vi "Vacuum Test - Step 5.vi"(7 "Step":i32, 8 "error in":errorcluster, 9 "Test Results In":T9, 10 "PAS In":T8 caption="Gas", 11 "Test Configuration":T1) -> (0 "error out":errorcluster, 1 "Test Results Out":T9, 2 "PAS Out":T8 caption="Gas", 3 "Test Configuration Out":T1)   [LabVIEW 2015]
uses:
  CAN Communication/PAS/Typedefs/Session Handle.ctl
  CAN Communication/PAS/PAS.lvclass
  Controls/Test Results.ctl
  Controls/Step Result.ctl
  Controls/Test Configuration.ctl
  Controls/Vacuum Test.ctl
  Controls/Test Timing.ctl
  Controls/Vaccum Thresholds.ctl
  Controls/Helium Test.ctl
  Controls/Helium Thresholds.ctl
  Controls/Functional Test.ctl
  CAN Communication/PAS/Typedefs/Valves.ctl
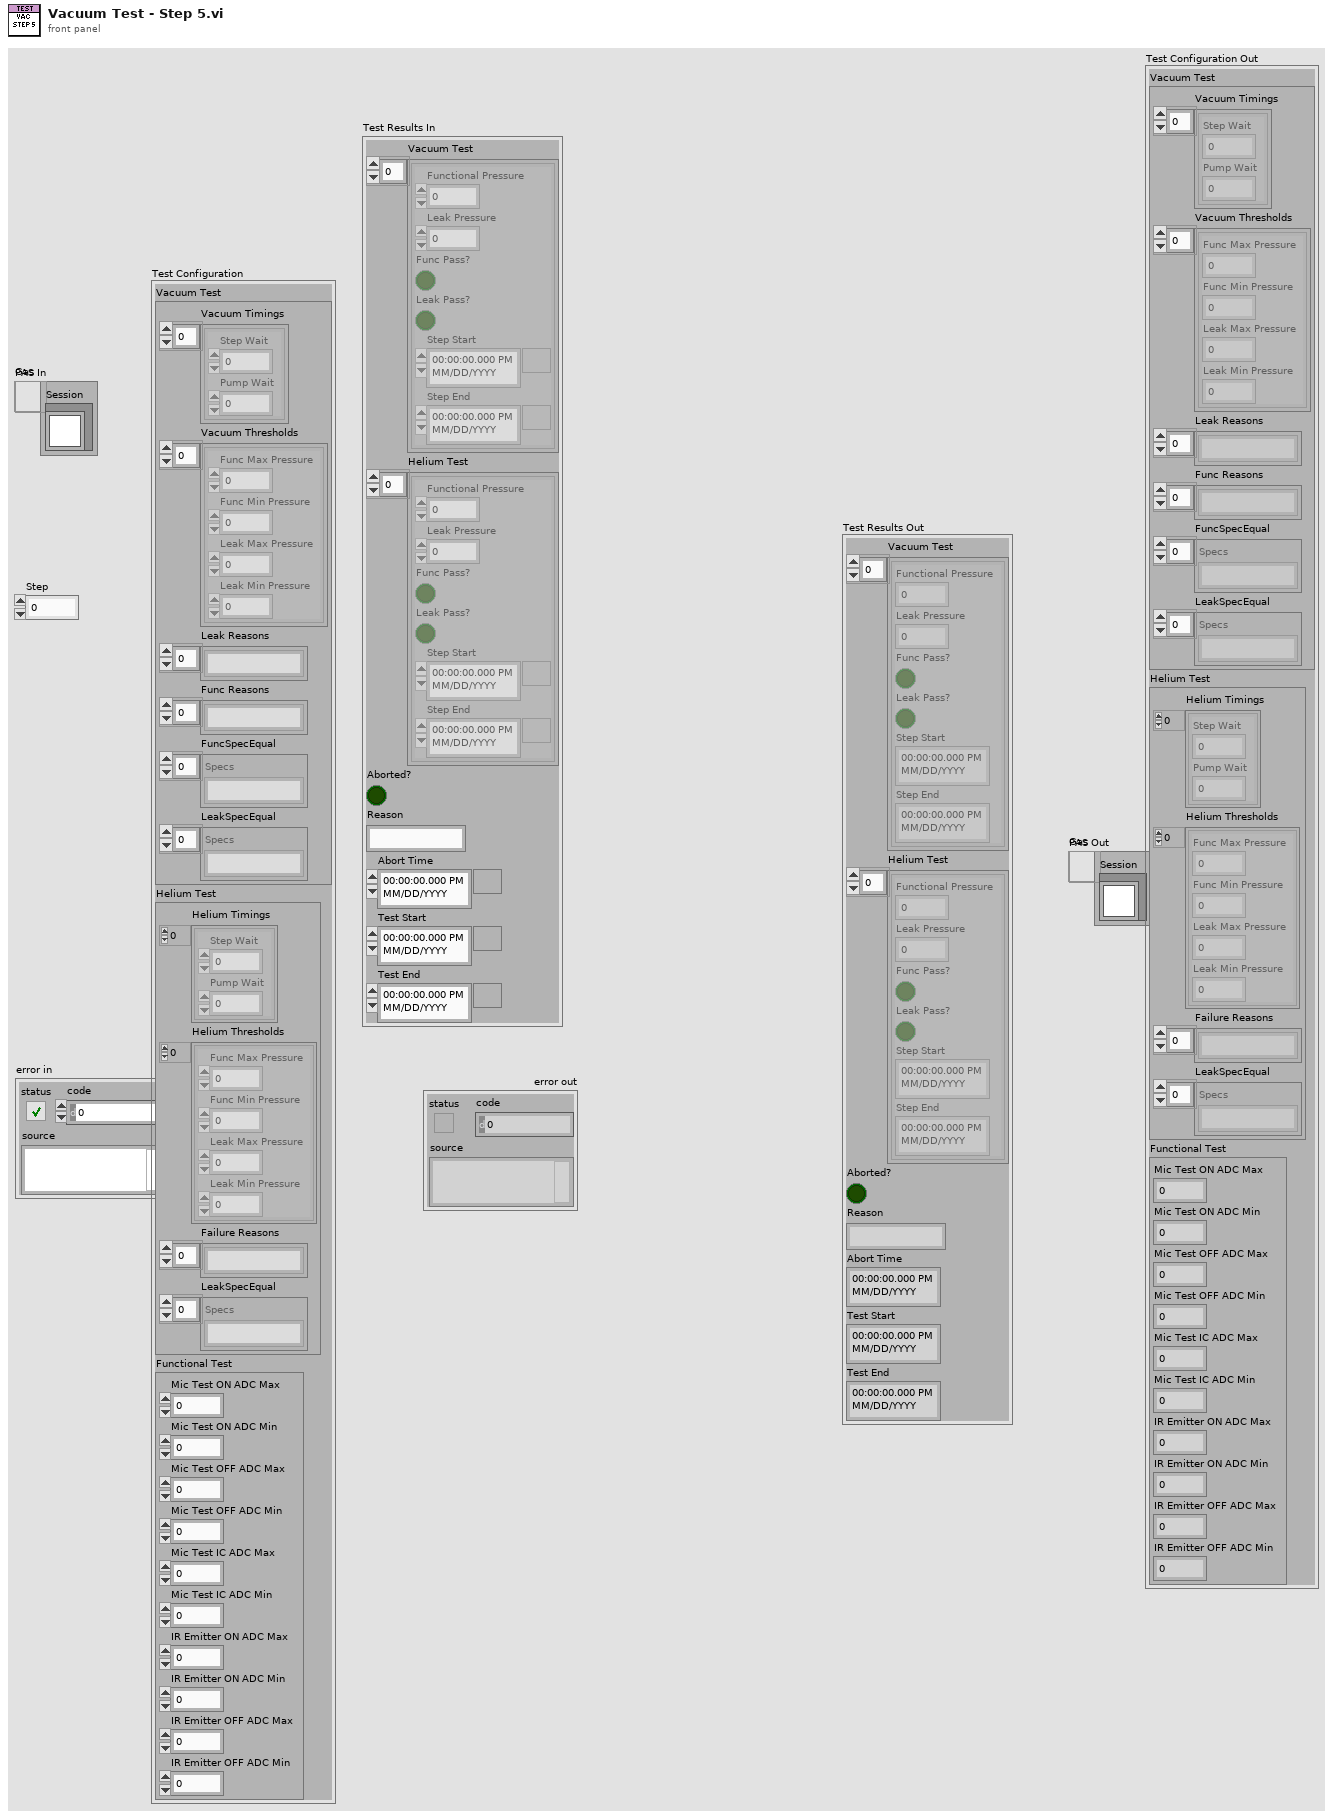
[diagram p1: front panel]
types:
  T1 = typedef "Test Configuration.ctl" = cluster{"Vacuum Test":T2, "Helium Test":T5, "Functional Test":T7}
  T2 = typedef "Vacuum Test.ctl" = cluster{"Vacuum Timings":T3[], "Vacuum Thresholds":T4[], "Leak Reasons":string[], "Func Reasons":string[], "FuncSpecEqual":string[], "LeakSpecEqual":string[]}
  T3 = typedef "Test Timing.ctl" = cluster{"Step Wait":dbl, "Pump Wait":dbl}
  T4 = typedef "Vaccum Thresholds.ctl" = cluster{"Func Max Pressure":dbl, "Func Min Pressure":dbl, "Leak Max Pressure":dbl, "Leak Min Pressure":dbl}
  T5 = typedef "Helium Test.ctl" = cluster{"Helium Timings":T3[], "Helium Thresholds":T6[], "Failure Reasons":string[], "LeakSpecEqual":string[]}
  T6 = typedef "Helium Thresholds.ctl" = cluster{"Func Max Pressure":dbl, "Func Min Pressure":dbl, "Leak Max Pressure":dbl, "Leak Min Pressure":dbl}
  T7 = typedef "Functional Test.ctl" = cluster{"Mic Test ON ADC Max":dbl, "Mic Test ON ADC Min":dbl, "Mic Test OFF ADC Max":dbl, "Mic Test OFF ADC Min":dbl, "Mic Test IC ADC Max":dbl, "Mic Test IC ADC Min":dbl, "IR Emitter ON ADC Max":dbl, "IR Emitter ON ADC Min":dbl, "IR Emitter OFF ADC Max":dbl, "IR Emitter OFF ADC Min":dbl}
  T8 = typedef "PAS.lvclass/Session Handle.ctl" = refnum<data-value>
  T9 = typedef "Test Results.ctl" = cluster{"Vacuum Test":T10[], "Helium Test":T10[], "Aborted?":bool, "Reason":string, "Abort Time":timestamp, "Test Start":timestamp, "Test End":timestamp}
  T10 = typedef "Step Result.ctl" = cluster{"Functional Pressure":dbl, "Leak Pressure":dbl, "Func Pass?":bool, "Leak Pass?":bool, "Step Start":timestamp, "Step End":timestamp}
  T11 = typedef "PAS.lvclass/Valves.ctl" = u16
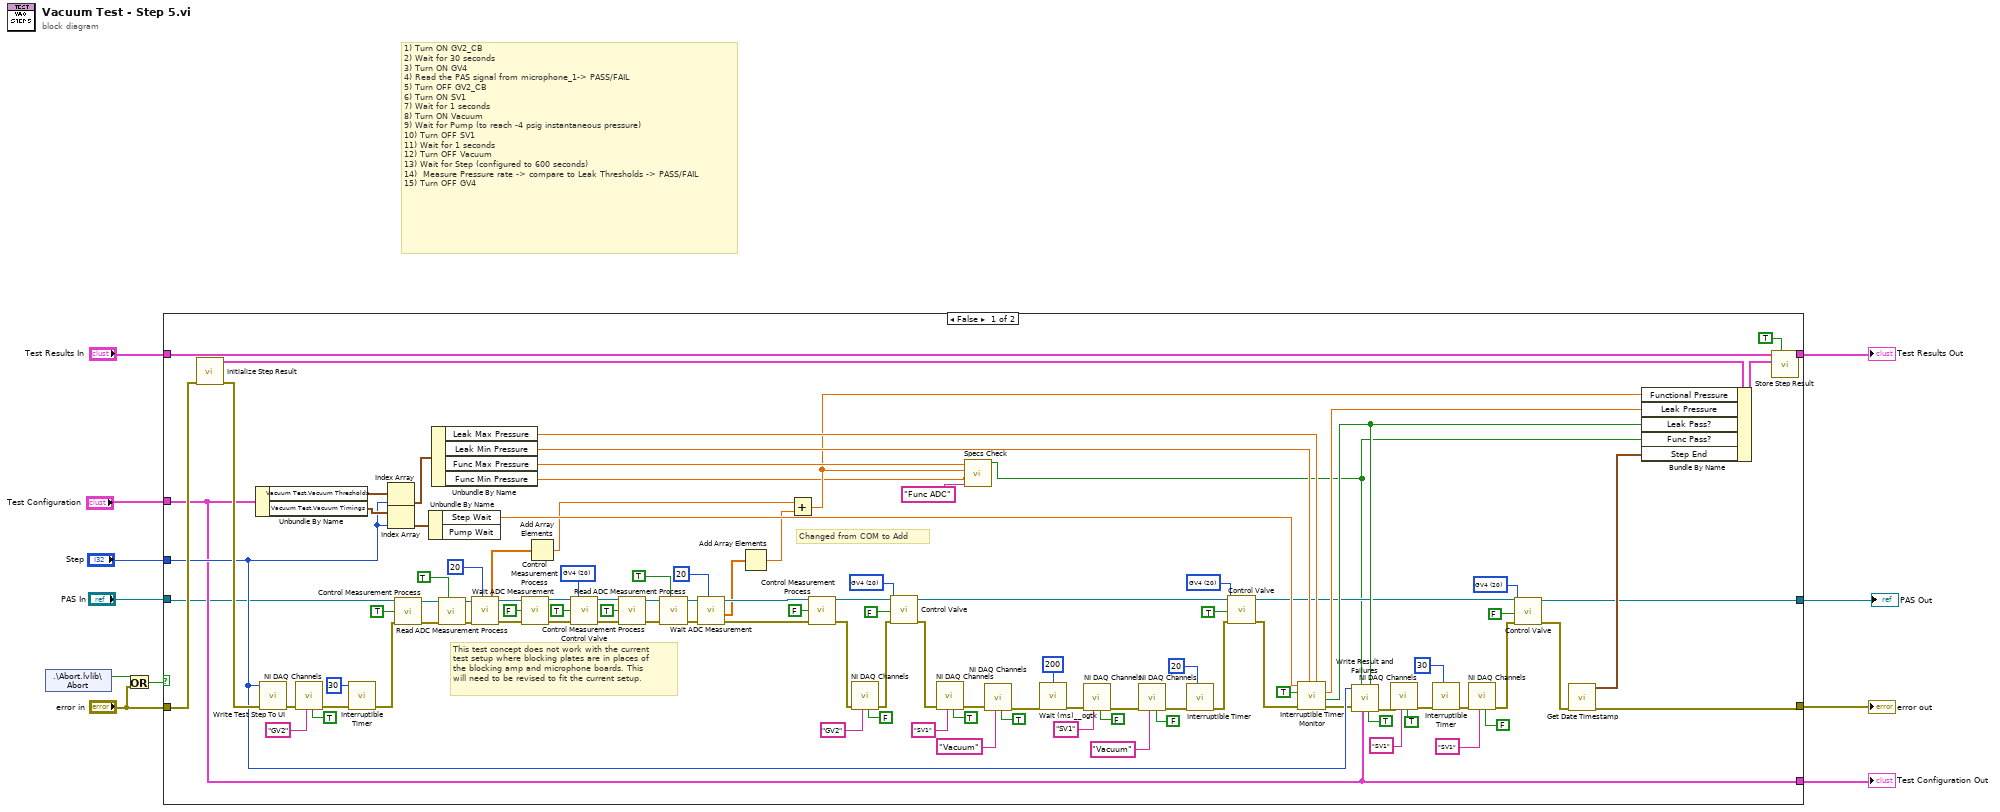
[diagram p0: block diagram]
diagram:
  # "1) Turn ON GV2_CB\n2) Wait for 30 seconds\n3) Turn ON GV4\n4) Read the PAS signal from microphone_1-> PASS/FAIL\n5) Turn OFF GV2_CB\n6) Turn ON SV1\n7) Wait for 1 seconds\n8) Turn ON Vacuum\n9) Wait for Pump (to reach -4 psig instantaneous pressure)\n10) Turn OFF SV1\n11) Wait for 1 seconds\n12) Turn OFF Vacuum\n13) Wait for Step (configured to 600 seconds)\n14)  Measure Pressure rate -> compare to Leak Thresholds -> PASS/FAIL\n15) Turn OFF GV4"
  n1 = shared-variable ".\\Abort.lvlib\\Abort"() -> (w10:bool)  [unwired: 1 in, 1 out]
  n2 = Or(x=w10, y="error in") -> (x .or. y?=w9:bool)
  n3 = case shown="False" w9 {
    tunnel: "error in" -> [w118 w121]
    tunnel: "Test Results In" -> [w115 w122]
    tunnel: [w116 w122] -> w7
    tunnel: [w58 w121] -> w6
    tunnel: "Test Configuration" -> [w99 w120]
    tunnel: "Step" -> [w106 _]
    tunnel: [w99 w120] -> w1
    tunnel: [w93 w119] -> w3
    tunnel: "PAS In" -> [w35 w119]
    frame False {
      w43 = T11 20 items=["GV1"=17, "GV2"=18, "GV3"=19, "GV4"=20] ("Valves")
      w65 = T11 20 items=["GV1"=17, "GV2"=18, "GV3"=19, "GV4"=20] ("Valves")
      w73 = T11 20 items=["GV1"=17, "GV2"=18, "GV3"=19, "GV4"=20] ("Valves")
      w95 = T11 20 items=["GV1"=17, "GV2"=18, "GV3"=19, "GV4"=20] ("Valves")
      # "Changed from COM to Add"
      # "This test concept does not work with the current\ntest setup where blocking plates are in places of\nthe blocking amp and microphone boards. This\nwill need to be revised to fit the current setup."
      n4 = call "Initialize Step Result.vi"("error in (no error)"=w118) -> ("error out"=w117:errorcluster, "New Step Result"=w114:T10)  [unwired: 8 in, 1 out]
      n5 = Unbundle By Name(w99) -> ("Vacuum Test.Vacuum Thresholds"=w111:T4[], "Vacuum Test.Vacuum Timings"=w110:T3[])
      n6 = call "Write Test Step To UI.vi"("error in (no error)"=w117, "Step"=w106) -> ("error out"=w104:errorcluster)  [unwired: 9 in]
      n7 = call "NI DAQ Channels.vi"("Control"=TRUE ("State"), "Channel"="GV2", "error in (no error)"=w104) -> ("error out"=w103:errorcluster)  [unwired: 7 in, 1 out]
      n8 = call "Interruptible Timer.vi"("error in (no error)"=w103, "Wait (s)"=30) -> ("error out"=w34:errorcluster)  [unwired: 7 in, 2 out]
      n9 = Index Array(array=w111, index=w106) -> (element=w107:T4)
      n10 = Index Array(array=w110, index=w106) -> (element=w109:T3)
      n11 = call "Control Measurement Process.vi"("Session Handle in"=w35, "Start?"=TRUE, "error in (no error)"=w34) -> ("Session Handle out"=w33:T8, "error out"=w32:errorcluster)  [unwired: 9 in, 2 out]
      n12 = Unbundle By Name(w109) -> ("Step Wait"=w79:dbl)  [unwired: 1 out]
      n13 = Unbundle By Name(w107) -> ("Leak Max Pressure"=w77:dbl, "Leak Min Pressure"=w78:dbl, "Func Max Pressure"=w17:dbl, "Func Min Pressure"=w15:dbl)
      n14 = call "Read ADC Measurement Process.vi"("Measurement Started?"=TRUE, "error in (no error)"=w32, "Session Handle in"=w33) -> ("error out"=w29:errorcluster, "Session Handle out"=w30:T8)  [unwired: 6 in, 1 out]
      n15 = call "Wait ADC Measurement.vi"("Wait (s)"=20, "error in (no error)"=w29, "Session Handle in"=w30) -> ("error out"=w47:errorcluster, "Array"=w27:dbl[], "Session Handle out"=w48:T8)  [unwired: 5 in, 1 out]
      n16 = call "Control Measurement Process.vi"("Session Handle in"=w48, "Start?"=FALSE, "error in (no error)"=w47) -> ("Session Handle out"=w45:T8, "error out"=w44:errorcluster)  [unwired: 9 in, 2 out]
      n17 = Add Array Elements(numeric array=w27) -> (sum=w12:dbl)
      n18 = call "Control Valve.vi"("Session Handle in"=w45, "Valves"=w43, "Energize?"=TRUE, "error in (no error)"=w44) -> ("Session Handle out"=w26:T8, "error out"=w25:errorcluster)  [unwired: 8 in, 2 out]
      n19 = call "Control Measurement Process.vi"("Session Handle in"=w26, "Start?"=TRUE, "error in (no error)"=w25) -> ("Session Handle out"=w24:T8, "error out"=w23:errorcluster)  [unwired: 9 in, 2 out]
      n20 = call "Read ADC Measurement Process.vi"("Measurement Started?"=TRUE, "error in (no error)"=w23, "Session Handle in"=w24) -> ("error out"=w21:errorcluster, "Session Handle out"=w22:T8)  [unwired: 6 in, 1 out]
      n21 = call "Wait ADC Measurement.vi"("Wait (s)"=20, "error in (no error)"=w21, "Session Handle in"=w22) -> ("error out"=w40:errorcluster, "Array"=w19:dbl[], "Session Handle out"=w41:T8)  [unwired: 5 in, 1 out]
      n22 = Add Array Elements(numeric array=w19) -> (sum=w13:dbl)
      n23 = Add(x=w12, y=w13) -> (x+y=w16:dbl)
      n24 = call "Control Measurement Process.vi"("Session Handle in"=w41, "Start?"=FALSE, "error in (no error)"=w40) -> ("Session Handle out"=w71:T8, "error out"=w91:errorcluster)  [unwired: 9 in, 2 out]
      n25 = call "NI DAQ Channels.vi"("Control"=FALSE ("State"), "Channel"="GV2", "error in (no error)"=w91) -> ("error out"=w70:errorcluster)  [unwired: 7 in, 1 out]
      n26 = call "Control Valve.vi"("Session Handle in"=w71, "Valves"=w73, "Energize?"=FALSE, "error in (no error)"=w70) -> ("Session Handle out"=w64:T8, "error out"=w69:errorcluster)  [unwired: 8 in, 2 out]
      n27 = call "NI DAQ Channels.vi"("Control"=TRUE ("State"), "Channel"="SV1", "error in (no error)"=w69) -> ("error out"=w90:errorcluster)  [unwired: 7 in, 1 out]
      n28 = call "Specs Check.vi"("parameter"="Func ADC", "lower limit"=w15, "x"=w16, "upper limit"=w17) -> ("In Range?"=w18:bool)  [unwired: 6 in, 1 out]
      n29 = call "NI DAQ Channels.vi"("Control"=TRUE ("State"), "Channel"="Vacuum", "error in (no error)"=w90) -> ("error out"=w89:errorcluster)  [unwired: 7 in, 1 out]
      n30 = call <userlib>:"Wait (ms)__ogtk.vi"("error in (no error)"=w89, "milliseconds to wait"=u32 200) -> ("error out"=w88:errorcluster)  [unwired: 8 in, 1 out]
      n31 = call "NI DAQ Channels.vi"("Control"=FALSE ("State"), "Channel"="SV1", "error in (no error)"=w88) -> ("error out"=w86:errorcluster)  [unwired: 7 in, 1 out]
      n32 = call "NI DAQ Channels.vi"("Control"=FALSE ("State"), "Channel"="Vacuum", "error in (no error)"=w86) -> ("error out"=w68:errorcluster)  [unwired: 7 in, 1 out]
      n33 = call "Interruptible Timer.vi"("error in (no error)"=w68, "Wait (s)"=20) -> ("error out"=w63:errorcluster)  [unwired: 7 in, 2 out]
      n34 = call "Control Valve.vi"("Session Handle in"=w64, "Valves"=w65, "Energize?"=TRUE, "error in (no error)"=w63) -> ("Session Handle out"=w61:T8, "error out"=w62:errorcluster)  [unwired: 8 in, 2 out]
      n35 = call "Interruptible Timer Monitor.vi"("Max"=w77, "Min"=w78, "error in (no error)"=w62, "Update UI?"=TRUE, "Wait (s)"=w79) -> ("error out"=w60:errorcluster, "In Range?"=w74:bool, "Leak Rate"=w76:dbl)  [unwired: 2 in, 2 out]
      n36 = call "Write Result and Failures.vi"("Vacuum?"=TRUE, "Leak"=w74, "Test Configuration"=w99, "Func"=w18, "error in (no error)"=w60, "Step"=w106) -> ("error out"=w59:errorcluster)  [unwired: 5 in]
      n37 = call "NI DAQ Channels.vi"("Control"=TRUE ("State"), "Channel"="SV1", "error in (no error)"=w59) -> ("error out"=w83:errorcluster)  [unwired: 7 in, 1 out]
      n38 = call "Interruptible Timer.vi"("error in (no error)"=w83, "Wait (s)"=30) -> ("error out"=w81:errorcluster)  [unwired: 7 in, 2 out]
      n39 = call "NI DAQ Channels.vi"("Control"=FALSE ("State"), "Channel"="SV1", "error in (no error)"=w81) -> ("error out"=w75:errorcluster)  [unwired: 7 in, 1 out]
      n40 = call "Control Valve.vi"("Session Handle in"=w61, "Valves"=w95, "Energize?"=FALSE, "error in (no error)"=w75) -> ("Session Handle out"=w93:T8, "error out"=w92:errorcluster)  [unwired: 8 in, 2 out]
      n41 = call "Get Date Timestamp.vi"("error in (no error)"=w92) -> ("error out"=w58:errorcluster, "current time"=w112:timestamp)  [unwired: 9 in]
      n42 = Bundle By Name(cluster=w114, "Functional Pressure"=w16, "Leak Pressure"=w76, "Leak Pass?"=w74, "Func Pass?"=w18, "Step End"=w112) -> (w113:T10)
      n43 = call "Store Step Result.vi"("Vacuum?"=TRUE, "Step Result"=w113, "Test Results In"=w115) -> ("Test Results Out"=w116:T9)  [unwired: 8 in]
    }
    frame True {
    }
  }
  "error out" <- w6
  "Test Results Out" <- w7
  "PAS Out" <- w3
  "Test Configuration Out" <- w1
